vi "just-drive-into-auto-zone Autonomous.vi"   [LabVIEW 2014]
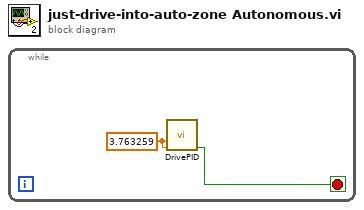
[diagram p0: block diagram]
diagram:
  n1 = while {
    stop <- w1 stop-if-true
    w2 = 3.763259 ("SetpointRight")
    n2 = call "DrivePID.vi"("SetpointRight"=w2, "SetpointLeft"=w2) -> ("Done"=w1:bool)  [unwired: 13 in]
  }
